vi "Object.vi"() -> ()   [LabVIEW 2017]
doc: "This example illustrates how to access private data members of an object."
uses:
  Example Class/Example Class.lvclass
  Example Class/Example Class.lvclass/Example Class.ctl
  57fc3f9c-a3a5-44be-bf17-76d2b860735a.vi
  a6d02755-27e1-4bf9-8589-1373b7bf1ffb.vi
  Example Class/Read Message.vi
  <vilib>/Utility/LVClass/Qualified Name Array To Single String.vi
  Composition/Composition.lvlib
panel:
  out "Message":string
  out "error out":errorcluster
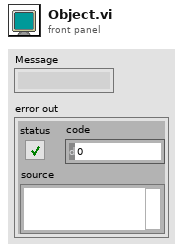
[diagram p1: front panel]
types:
  T1 = cluster{"Major":u16, "Minor":u16, "Fix":u16, "Build":u16}[]
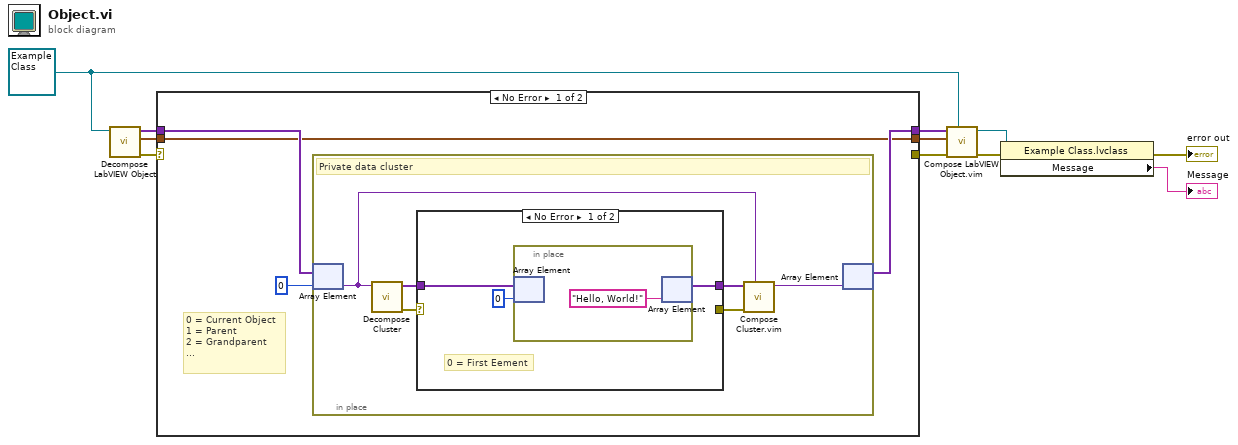
[diagram p0: block diagram]
diagram:
  w11 = refnum<class "Example Class.lvclass"> refnum ("Example Class.lvclass")
  n1 = call "Decompose LabVIEW Object.vi"("LabVIEW Object"=w11) -> ("error out"=w8:errorcluster, "Library Versions"=w7:T1, "Private Data Clusters"=w10:variant[])  [unwired: 7 in, 1 out]
  n2 = case shown="No Error" w8 {
    selector: w8 -> [_ w28]
    tunnel: w10 -> [w15 w29]
    tunnel: [w13 w29] -> w9
    tunnel: w7 -> [w12 w30]
    tunnel: [w12 w30] -> w6
    tunnel: [_ w28] -> w5
    frame No Error {
      # "0 = Current Object\n1 = Parent\n2 = Grandparent\n..."
      n3 = in-place {
        # "Private data cluster"
        n4 = in-place-array #1(w15, 0) -> (w20:variant)
        n5 = call "Decompose Cluster.vi"("Variant Cluster"=w20) -> ("error out"=w17:errorcluster, "Cluster Elements"=w19:variant[])  [unwired: 9 in]
        n6 = case shown="No Error" w17 {
          selector: w17 -> [_ w27]
          tunnel: w19 -> [w24 w26]
          tunnel: [w23 w26] -> w18
          tunnel: [_ w27] -> w16
          frame No Error {
            # "0 = First Eement"
            n7 = in-place {
              n8 = in-place-array #2(w24, 0) -> ()  [unwired: 1 out]
              n9 = in-place-array #2("Hello, World!") -> (w23:variant[])  [unwired: 1 out]
            }
          }
          frame Error {
          }
        }
        n10 = call "Compose Cluster.vim"("Type"=w20, "error in"=w16, "Elements"=w18) -> ("Cluster"=w21:variant)  [unwired: 7 in, 1 out]
        n11 = in-place-array #1(w21) -> (w13:variant[])  [unwired: 1 out]
      }
    }
    frame Error {
    }
  }
  n12 = call "Compose LabVIEW Object.vim"("Type"=w11, "error in (no error)"=w5, "Library Versions"=w6, "Private Data Clusters"=w9) -> ("error out"=w4:errorcluster, "LabVIEW Object"=w2:refnum<class "Example Class.lvclass">)  [unwired: 6 in]
  n13 = property class="Example Class.lvclass"(reference=w2, error in=w4) -> (error out=→"error out":errorcluster, "Message"=→"Message":string)  [unwired: 1 out]
